vi "RS_SMBV100A_RequestWaypoints.vi"(0 "DriverConnect in":T1={"InterfaceType"=enum."VISA", "OpenedSession"="", "InterfaceSettings"={"Interface"=enum."RS232", "EOS 4 read"=enum."LF (\\n)", "EOS 4 write"=enum."LF (\\n)", "TMO, ms"=10000, "Sett"=variant(cluster{"Baud Rate":u32, "Data Bits":u16, "Parity":u16, "Stop Bits":u16, "Flow Control":u16, "Eho":bool} {"Baud Rate"=75, "Data Bits"=0, "Parity"=0, "Stop Bits"=0, "Flow Control"=0, "Eho"=FALSE})}}, 1 "scenario time, c":dbl, 11 "Error In":errorcluster, 12 "BASEBAND":string="GPS", 13 "Scenario in":string="****************************** MOVEMENT FILE ******************************\nRESOLUTION: 50\nREFERENCE: 11.583333,48.150,500\nSTART: 0, 0, 0, 10\nSTAY: 10000\nLINE: 200, 0, 0\nLINE: 100, 0, 19,6\nLINE: 600, 0, 0\nLINE: 100, 0, -19,6\nARC: 0, 0, 180\nLINE: -200, 0, 0\nLINE: -100, 0, 19,6\nLINE: -600, 0, 0\nLINE: 100, 0, -19,6\nARC: 0, 0, -180") -> (3 "Dynam waypoints":T6 {"Time" format="%<%.3X>T"; "Speed" format="%#.10g"; "Heigth" format="%#.10g"; "Longitude" format="%#.10g"; "Latitude" format="%#.10g"}, 4 "DriverConnect out":T1={"InterfaceType"=enum."VISA", "OpenedSession"="", "InterfaceSettings"={"Interface"=enum."RS232", "EOS 4 read"=enum."LF (\\n)", "EOS 4 write"=enum."LF (\\n)", "TMO, ms"=10000, "Sett"=variant(cluster{"Baud Rate":u32, "Data Bits":u16, "Parity":u16, "Stop Bits":u16, "Flow Control":u16, "Eho":bool} {"Baud Rate"=75, "Data Bits"=0, "Parity"=0, "Stop Bits"=0, "Flow Control"=0, "Eho"=FALSE})}}, 14 "Waypoints, txt":string="R&S_SMBV100A", 15 "Error Out":errorcluster)   [LabVIEW 2018]
uses:
  RS_SMBV100A_DynamWaypoints.ctl
  RS_SMBV100A_DynamWaypoint.ctl
  MOKO_LabViewLibrary/MokoLowLevel/MokoLowLovelControl/MLLC_ConnectCluster.ctl
  MOKO_LabViewLibrary/MokoLowLevel/MokoLowLovelControl/MLLC_InterfaceType.ctl
  MOKO_LabViewLibrary/MokoLowLevel/MokoLowLovelControl/MLLC_OpenedSession.ctl
  MOKO_LabViewLibrary/MokoLowLevel/MokoLowLovelControl/MLLC_InterfaceSettings.ctl
  MOKO_LabViewLibrary/MokoLowLevel/MokoLowLovelControl/MLLC_InterfaceKind.ctl
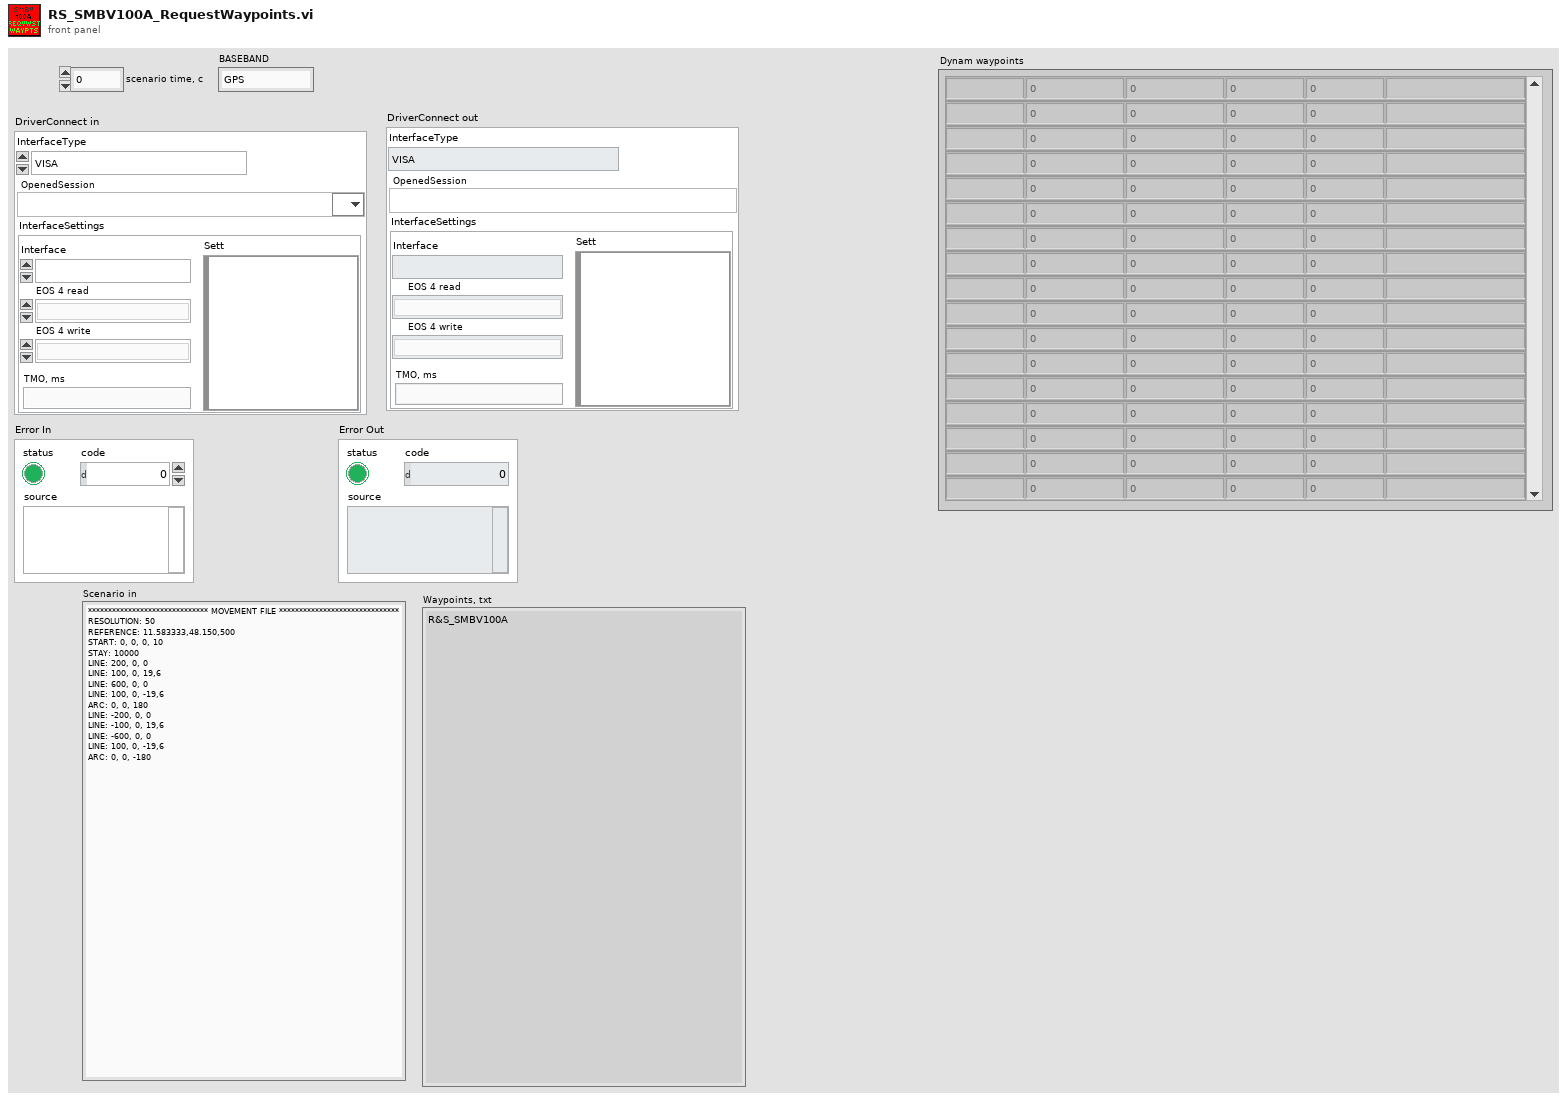
[diagram p1: front panel]
types:
  T1 = typedef "MLLC_ConnectCluster.ctl" = cluster{"InterfaceType":T2, "OpenedSession":T3, "InterfaceSettings":T4}
  T2 = typedef "MLLC_InterfaceType.ctl" = enum16{"VISA", "Prologix USB-GPIB"}
  T3 = typedef "MLLC_OpenedSession.ctl" = refnum<visa-resource-name>
  T4 = typedef "MLLC_InterfaceSettings.ctl" = cluster{"Interface":T5, "EOS 4 read":enum16{"Default (=EOS 4 write)", "CR (\\r)", "LF (\\n)", "None"}, "EOS 4 write":enum16{"CR+LF (\\r\\n)", "CR (\\r)", "LF (\\n)", "None"}, "TMO, ms":i32, "Sett":variant}
  T5 = typedef "MLLC_InterfaceKind.ctl" = enum16{"RS232", "GPIB", "USB", "Ethernet", "another"}
  T6 = typedef "RS_SMBV100A_DynamWaypoints.ctl" = T7[]
  T7 = typedef "RS_SMBV100A_DynamWaypoint.ctl" = cluster{"Time":timestamp, "Latitude":ext, "Longitude":ext, "Heigth":dbl, "Speed":dbl, "Scenario":string}
  T8 = typedef "RS_SMBV100A_ScenarioInfo.ctl" = cluster{"RESOLUTION":dbl, "Duration, s":dbl, "scenario lines":T9[]}
  T9 = typedef "RS_SMBV100A_ScenarioLineInfo.ctl" = cluster{"Type":string, "Start time, s":dbl, "Start speed, m\\s":dbl, "Acceleration, m\\s2":dbl, "Duration, s":dbl, "Stop time, s":dbl, "Scenario Name":string}
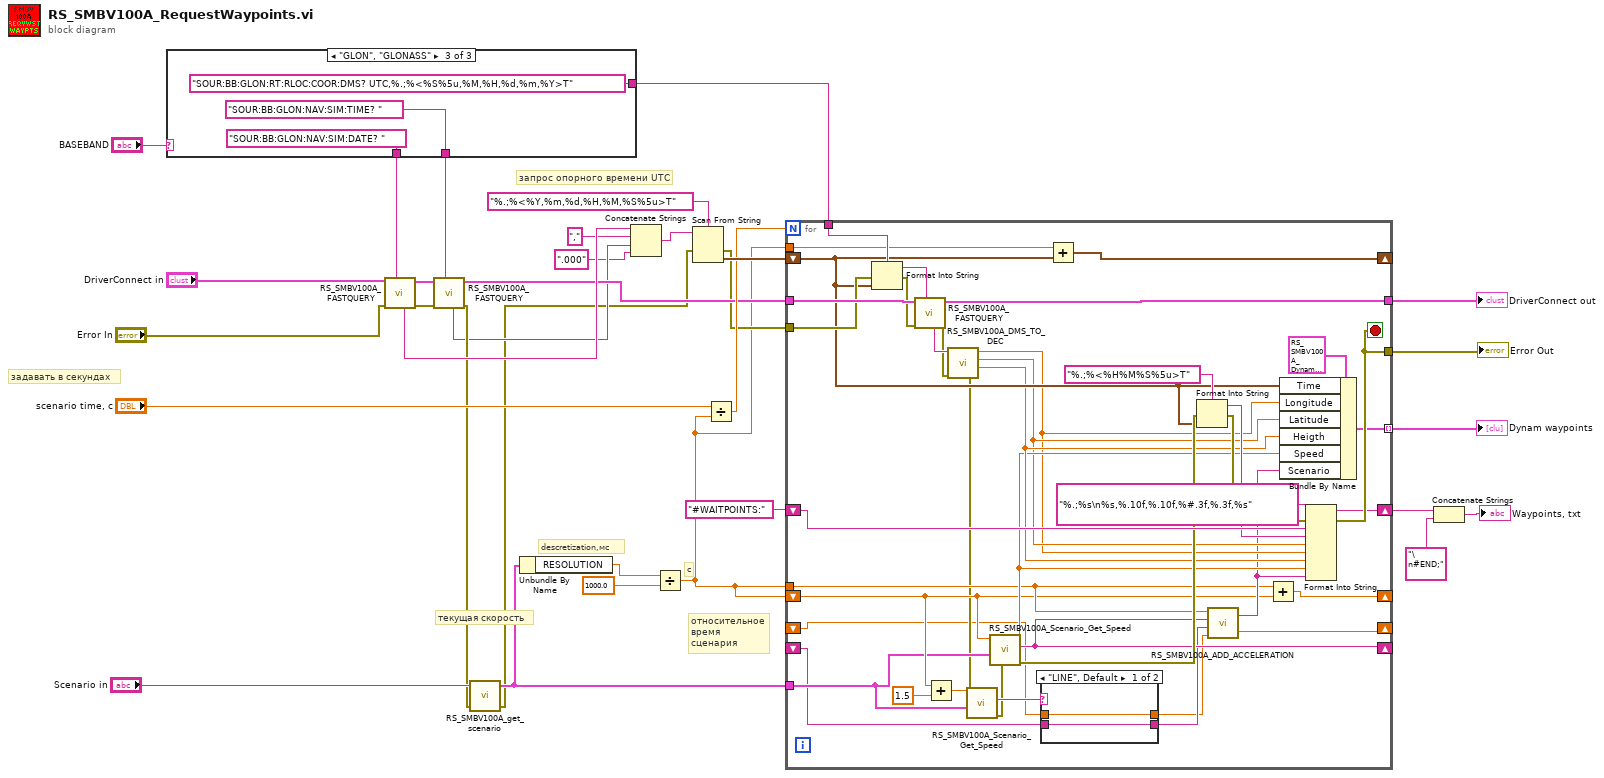
[diagram p0: block diagram]
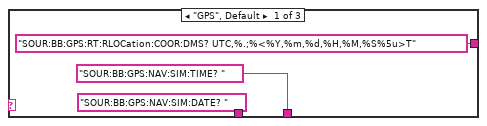
[diagram p2: hidden frame]
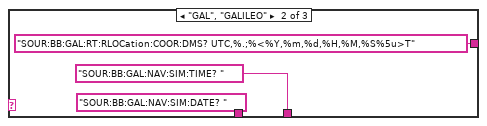
[diagram p3: hidden frame]
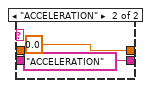
[diagram p4: hidden frame]
diagram:
  # "с"
  # "descretization,мс"
  # "текущая скорость"
  # "относительное\nвремя \nсценария"
  # "запрос опорного времени UTC"
  # "задавать в секундах"
  n1 = case shown="\"GLON\", \"GLONASS\"" "BASEBAND" {
    tunnel: ["SOUR:BB:GPS:NAV:SIM:DATE? " ("regular expression") "SOUR:BB:GAL:NAV:SIM:DATE? " ("regular expression") "SOUR:BB:GLON:NAV:SIM:DATE? " ("regular expression")] -> w33
    tunnel: ["SOUR:BB:GPS:NAV:SIM:TIME? " ("regular expression") "SOUR:BB:GAL:NAV:SIM:TIME? " ("regular expression") "SOUR:BB:GLON:NAV:SIM:TIME? " ("regular expression")] -> w32
    tunnel: ["SOUR:BB:GPS:RT:RLOCation:COOR:DMS? UTC,%.;%<%Y,%m,%d,%H,%M,%S%5u>T" ("format string") "SOUR:BB:GAL:RT:RLOCation:COOR:DMS? UTC,%.;%<%Y,%m,%d,%H,%M,%S%5u>T" ("format string") "SOUR:BB:GLON:RT:RLOC:COOR:DMS? UTC,%.;%<%S%5u,%M,%H,%d,%m,%Y>T" ("format string")] -> w16
    frame "GPS", Default {
    }
    frame "GAL", "GALILEO" {
    }
    frame "GLON", "GLONASS" {
    }
  }
  n2 = call "RS_SMBV100A_FASTQUERY.vi"("input"=w33, "Error In"="Error In", "DriverConnect in"="DriverConnect in") -> ("Error Out"=w30:errorcluster, "DriverConnect out"=w31:T1, "output"=w28:string)  [unwired: 6 in]
  n3 = call "RS_SMBV100A_FASTQUERY.vi"("input"=w32, "Error In"=w30, "DriverConnect in"=w31) -> ("Error Out"=w21:errorcluster, "DriverConnect out"=w23:T1, "output"=w15:string)  [unwired: 6 in]
  n4 = call "RS_SMBV100A_get_scenario.vi"("error in"=w21, "Scenario in"="Scenario in") -> ("error out"=w13:errorcluster, "Scenario info"=w20:T8)  [unwired: 2 in]
  n5 = Unbundle By Name(w20) -> ("RESOLUTION"=w18:dbl)
  n6 = Concatenate Strings(w28, "," ("format string"), w15, ".000" ("format string")) -> (w27:string)
  n7 = Divide(x=w18, y=1000.0) -> (x/y=w5:dbl)
  n8 = Scan From String(format string="%.;%<%Y,%m,%d,%H,%M,%S%5u>T", input string=w27, error in=w13) -> (error out=w12:errorcluster, output 1=w25:timestamp)  [unwired: 2 in, 2 out]
  n9 = Divide(x="scenario time, c", y=w5) -> (x/y=w24:dbl)
  n10 = for {
    N: w24 -> [_]
    shift-right: [w68] -> _
    shift-left: w25 -> [w63]
    tunnel: w16 -> [w83]
    tunnel: w23 -> [w79]
    tunnel: w12 -> [w78]
    tunnel: [w74] -> w3
    tunnel: [w76] -> w1
    shift-right: [w73] -> w7
    shift-left: "#WAITPOINTS:" -> [w71]
    tunnel: w5 -> [w69]
    shift-right: [w67] -> _
    shift-left: w5 -> [w53]
    tunnel: w5 -> [w54]
    tunnel: w20 -> [w50]
    tunnel: [w62] -> w8 mode=indexing
    shift-right: [w56] -> _
    shift-left: _ -> [w46]
    shift-right: [w55] -> _
    shift-left: _ -> [w44]
    stop <- w74 stop-if-true
    n11 = Format Into String(format string=w83, error in=w78, w63) -> (resulting string=w80:string, error out=w77:errorcluster)  [unwired: 1 in]
    n12 = call "RS_SMBV100A_FASTQUERY.vi"("input"=w80, "Error In"=w77, "DriverConnect in"=w79) -> ("Error Out"=w81:errorcluster, "DriverConnect out"=w76:T1, "output"=w82:string)  [unwired: 6 in]
    n13 = Add(x=w53, y=1.5) -> (x+y=w51:dbl)
    n14 = call "RS_SMBV100A_DMS_TO_DEC.vi"("error in"=w81, "DMS"=w82) -> ("error out"=w48:errorcluster, "hig"=w61:dbl, "lon"=w59:dbl, "lat"=w58:dbl)  [unwired: 6 in]
    n15 = call "RS_SMBV100A_Scenario_Get_Speed.vi"("error in"=w48, "Scenario info in"=w50, "Current Scenario Time, s"=w51) -> ("error out"=w47:errorcluster, "Scenario Name"=w49:string)  [unwired: 5 in, 2 out]
    n16 = call "RS_SMBV100A_Scenario_Get_Speed.vi"("error in"=w47, "Scenario info in"=w50, "Current Scenario Time, s"=w53) -> ("error out"=w66:errorcluster, "Scenario Name"=w56:string, "Speed, m\\s"=w60:dbl)  [unwired: 5 in, 1 out]
    n17 = case shown="\"LINE\", Default" w49 {
      tunnel: w46 -> [w85 _]
      tunnel: [w85 "ACCELERATION"] -> w45
      tunnel: w44 -> [w84 _]
      tunnel: [w84 0.0 ("y")] -> w43
      frame "LINE", Default {
      }
      frame "ACCELERATION" {
      }
    }
    n18 = Add(x=w69, y=w63) -> (x+y=w68:timestamp)
    n19 = Format Into String(format string="%.;%<%H%M%S%5u>T", error in=w66, w63) -> (resulting string=w70:string, error out=w65:errorcluster)  [unwired: 1 in]
    n20 = call "RS_SMBV100A_ADD_ACCELERATION.vi"("COUNT IN"=w43, "Scenario Name Previous"=w45, "Scenario Name New in"=w56, "RESOLUTION"=w54) -> ("COUNT OUT"=w55:dbl, "Scenario Name New out"=w57:string)
    n21 = Add(x=w54, y=w53) -> (x+y=w67:dbl)
    n22 = Bundle By Name(cluster=T7 {"Time"=timestamp(0 s since 1904-01-01), "Latitude"=0.0, "Longitude"=0.0, "Heigth"=0.0, "Speed"=0.0, "Scenario"=""} ("Cluster"), "Time"=w63, "Longitude"=w58, "Latitude"=w59, "Heigth"=w61, "Speed"=w60, "Scenario"=w57) -> (w62:T7)
    n23 = Format Into String(format string="%.;%s\n%s,%.10f,%.10f,%#.3f,%.3f,%s", error in=w65, w71, w70, w59, w58, w61, w60, w57) -> (resulting string=w73:string, error out=w74:errorcluster)  [unwired: 1 in]
  }
  "Dynam waypoints" <- w8
  "Error Out" <- w3
  "DriverConnect out" <- w1
  n24 = Concatenate Strings(w7, "\n#END;" ("regular expression")) -> (→"Waypoints, txt":string)
